vi "FileNames.vi"(5 "# Elements":i32=5, 6 "Plane":i32, 7 "Digits":i32=3, 8 "Dig Config":i32, 9 "Xmit Ring":i32, 10 "Scan Name":string, 11 "2-D motor":bool) -> (1 "RCV 1 File Name":string, 2 "Crate File Names":string[](array[string]), 3 "All files":string[](array[string]))   [LabVIEW 2022 SP3]
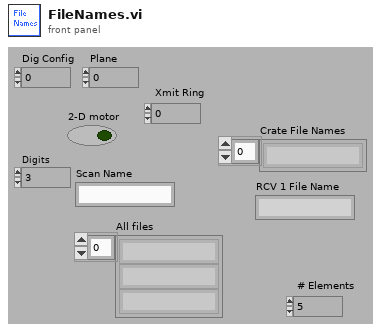
[diagram p1: front panel]
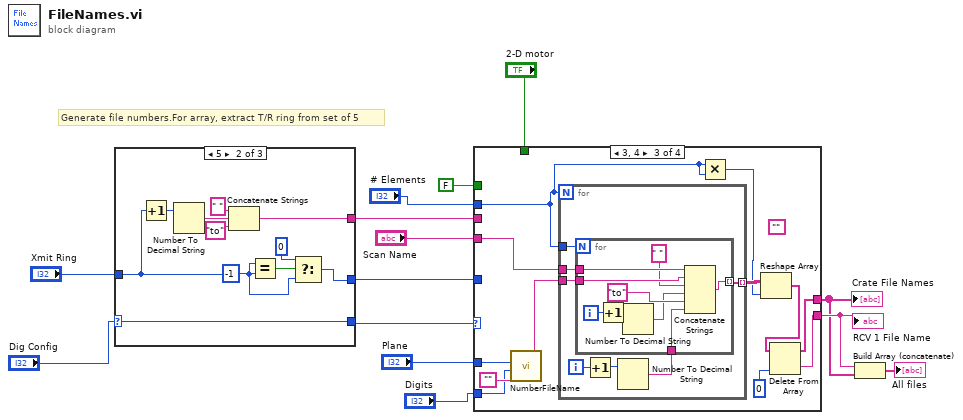
[diagram p0: block diagram]
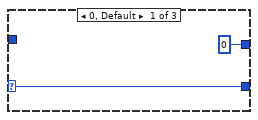
[diagram p2: hidden frame]
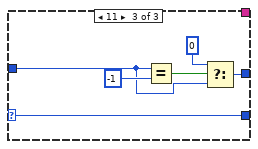
[diagram p3: hidden frame]
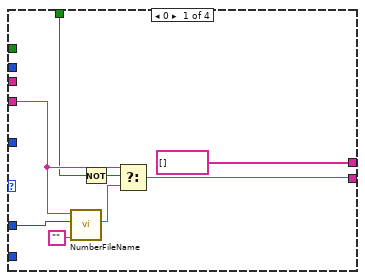
[diagram p4: hidden frame]
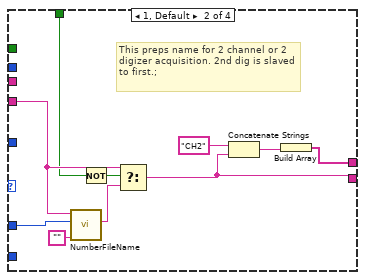
[diagram p5: hidden frame]
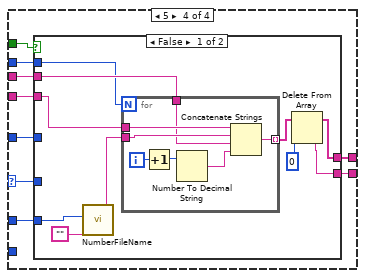
[diagram p6: hidden frame]
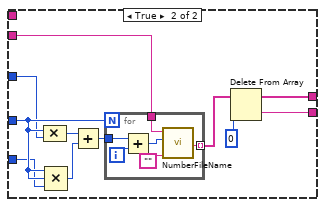
[diagram p7: hidden frame]
diagram:
  # "Generate file numbers.For array, extract T/R ring from set of 5"
  n1 = case shown="5" "Dig Config" {
    selector: "Dig Config" -> [w15 w23 w28]
    tunnel: "Xmit Ring" -> [_ w20 w31]
    tunnel: [0 w24 w29] -> w11
    tunnel: [w15 w23 w28] -> w13
    tunnel: [_ w18 _] -> w9
    frame 0, Default {
    }
    frame 5 {
      n2 = Increment(x=w20) -> (x+1=w17:i32)
      n3 = Number To Decimal String(number=w17) -> (decimal integer string=w19:string)  [unwired: 1 out]
      n4 = Concatenate Strings(" ", w19, "to") -> (w18:string)
      n5 = Equal?(x=w20, y=-1) -> (x = y?=w27:bool)
      n6 = Select(t=0, s=w27, f=w20) -> (s? t:f=w24:i32)
    }
    frame 11 {
      n7 = Equal?(x=w31, y=-1) -> (x = y?=w33:bool)
      n8 = Select(t=0, s=w33, f=w31) -> (s? t:f=w29:i32)
    }
  }
  n9 = case shown="3, 4" w13 {
    selector: w13 -> [_ _ _ w85]
    tunnel: "Scan Name" -> [w39 w50 w63 w88]
    tunnel: w11 -> [_ _ _ w84]
    tunnel: [w37 w42 w56 w87] -> w8
    tunnel: [string[] [] w44 w57 w86] -> w7
    tunnel: "Plane" -> [w34 w46 w62 w83]
    tunnel: "2-D motor" -> [w36 w48 _ _]
    tunnel: FALSE -> [_ _ _ w82]
    tunnel: w9 -> [_ _ _ w81]
    tunnel: "Digits" -> [_ _ w54 _]
    tunnel: "# Elements" -> [_ _ w53 w80]
    frame 0 {
      n10 = call "NumberFileName.vi"("String"="", "File number"=w34, "file name"=w39) -> ("Numbered File"=w40:string)  [unwired: 1 in]
      n11 = Not(x=w36) -> (.not. x?=w35:bool)
      n12 = Select(t=w39, s=w35, f=w40) -> (s? t:f=w37:string)
    }
    frame 1, Default {
      # "This preps name for 2 channel or 2 digizer acquisition. 2nd dig is slaved to first.;"
      n13 = call "NumberFileName.vi"("String"="", "File number"=w46, "file name"=w50) -> ("Numbered File"=w51:string)  [unwired: 1 in]
      n14 = Not(x=w48) -> (.not. x?=w47:bool)
      n15 = Select(t=w50, s=w47, f=w51) -> (s? t:f=w42:string)
      n16 = Concatenate Strings("CH2" ("string"), w42) -> (w45:string)
      n17 = Build Array(w45) -> (w44:string[])
    }
    frame 3, 4 {
      (unwired) ""
      n18 = call "NumberFileName.vi"("String"="", "Digits"=w54, "File number"=w62) -> ("Numbered File"=w59:string)  [unwired: 1 in]
      n19 = for {
        N: w53 -> [_]
        tunnel: w63 -> [w70]
        tunnel: [w69] -> w60 mode=indexing
        tunnel: w53 -> [w68]
        tunnel: w59 -> [w65]
        i -> [w66]
        n20 = Increment(x=w66) -> (x+1=w67:i32)
        n21 = Number To Decimal String(number=w67) -> (decimal integer string=w64:string)  [unwired: 1 out]
        n22 = for {
          N: w68 -> [_]
          tunnel: w70 -> [w79]
          tunnel: [w78] -> w69 mode=indexing
          tunnel: w65 -> [w75]
          tunnel: w64 -> [w71]
          i -> [w76]
          n23 = Increment(x=w76) -> (x+1=w77:i32)
          n24 = Number To Decimal String(number=w77) -> (decimal integer string=w72:string)  [unwired: 1 out]
          n25 = Concatenate Strings(w79, w75, " ", w72, "to", w71) -> (w78:string)
        }
      }
      n26 = Multiply(x=w53, y=w53) -> (x*y=w52:i32)
      n27 = Reshape Array(w60, w52) -> (w58:string[])
      n28 = Delete From Array(array=w58, index=0) -> (deleted portion=w56:string, array with subset deleted=w57:string[])  [unwired: 1 in]
    }
    frame 5 {
      n29 = case shown="False" w82 {
        tunnel: w88 -> [w96 w116]
        tunnel: [w90 w114] -> w87
        tunnel: [w91 w113] -> w86
        tunnel: w85 -> [_ w111]
        tunnel: w84 -> [_ w108]
        tunnel: w83 -> [w97 w107]
        tunnel: w81 -> [w94 _]
        tunnel: w80 -> [w89 _]
        frame False {
          n30 = call "NumberFileName.vi"("String"="", "File number"=w97) -> ("Numbered File"=w95:string)  [unwired: 2 in]
          n31 = for {
            N: w89 -> [_]
            tunnel: w96 -> [w104]
            tunnel: w95 -> [w103]
            tunnel: w94 -> [w102]
            tunnel: [w101] -> w92 mode=indexing
            i -> [w99]
            n32 = Increment(x=w99) -> (x+1=w100:i32)
            n33 = Number To Decimal String(number=w100) -> (decimal integer string=w105:string)  [unwired: 1 out]
            n34 = Concatenate Strings(w104, w103, w102, w105) -> (w101:string)
          }
          n35 = Delete From Array(array=w92, index=0) -> (deleted portion=w90:string, array with subset deleted=w91:string[])  [unwired: 1 in]
        }
        frame True {
          n36 = Compound Arithmetic op=MULTIPLY(w111, w108) -> (w109:i32)
          n37 = Compound Arithmetic op=MULTIPLY(w111, w111, w107) -> (w112:i32)
          n38 = Add(x=w109, y=w112) -> (x+y=w110:i32)
          n39 = for {
            N: w111 -> [_]
            tunnel: w110 -> [w121]
            tunnel: w116 -> [w119]
            tunnel: [w118] -> w115 mode=indexing
            i -> [w122]
            n40 = Add(x=w121, y=w122) -> (x+y=w120:i32)
            n41 = call "NumberFileName.vi"("String"="", "File number"=w120, "file name"=w119) -> ("Numbered File"=w118:string)  [unwired: 1 in]
          }
          n42 = Delete From Array(array=w115, index=0) -> (deleted portion=w114:string, array with subset deleted=w113:string[])  [unwired: 1 in]
        }
      }
    }
  }
  "Crate File Names" <- w7
  "RCV 1 File Name" <- w8
  n43 = Build Array (concatenate)(w8, w7) -> (→"All files":string[])
